vi "p2.vi"() -> ()   [LabVIEW 2023, in "d13.lvlib"]
uses:
  d13.lvlib
  AOC/AOC.lvlib
panel:
  out "XY Graph":cluster{i32, i32}[](graph)
  in  "Example":string="#.##..##.\n..#.##.#.\n##......#\n##......#\n..#.##.#.\n..##..##.\n#.#.##.#.\n\n#...##..#\n#....#..#\n..##..###\n#####.##.\n#####.##.\n..##..###\n#....#..#"
  in  "Example":bool=TRUE
  out "Answer":u64=5675
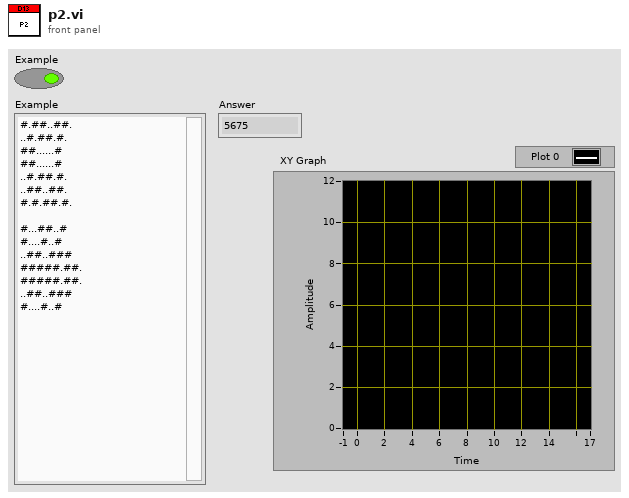
[diagram p1: front panel]
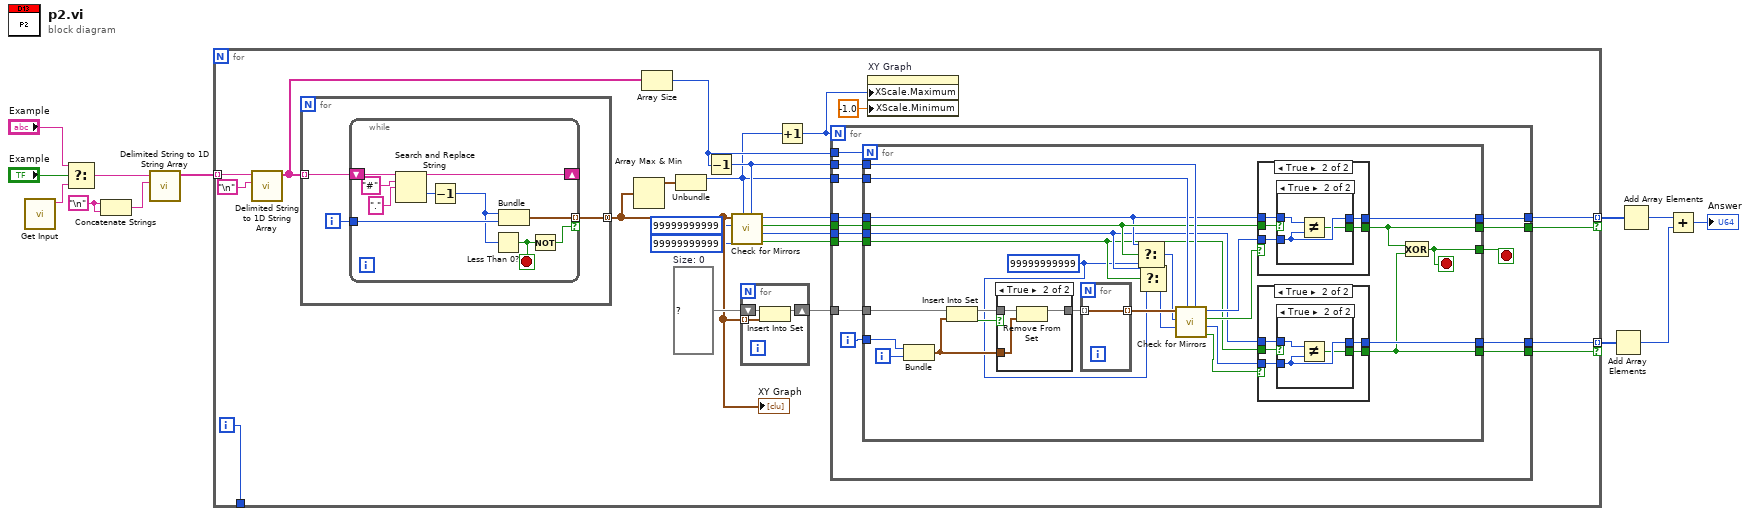
[diagram p0: block diagram]
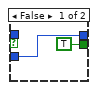
[diagram p3: hidden frame]
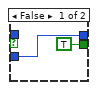
[diagram p5: hidden frame]
diagram:
  w5 = "\n"
  n1 = call "Get Input.vi"() -> ("Input"=w12:string)  [unwired: 11 in]
  n2 = Select(t="Example", s="Example", f=w12) -> (s? t:f=w8:string)
  n3 = Concatenate Strings(w5, w5) -> (w6:string)
  n4 = call <vilib>:"Delimited String to 1D String Array.vi"("delimiter"=w6, "delimited string"=w8) -> ("string array"=w7:string[])  [unwired: 9 in]
  n5 = for {
    tunnel: w7 -> [w35] mode=indexing
    tunnel: [w23] -> w9 mode=indexing if=w20
    tunnel: [w24] -> w4 mode=indexing if=w19
    tunnel: [w18] -> _
    i -> [w18]
    w31 = set{cluster{i32, i32}} {}  # Size: 0
    n6 = call <vilib>:"Delimited String to 1D String Array.vi"("delimiter"="\n", "delimited string"=w35) -> ("string array"=w32:string[])  [unwired: 9 in]
    n7 = for {
      tunnel: w32 -> [w110] mode=indexing
      tunnel: [w109] -> w17 mode=concatenating
      i -> [w108]
      n8 = while {
        tunnel: [w120] -> w109 mode=indexing if=w117
        tunnel: w108 -> [w119]
        shift-right: [w115] -> _
        shift-left: w110 -> [w116]
        stop <- w118 stop-if-true
        n9 = Search and Replace String(input string=w116, search string="#" ("search string/char (-)"), replace string="." ("replace string (\"\")")) -> (result string=w115:string, offset past replacement=w113:i32)  [unwired: 5 in, 2 out]
        n10 = Decrement(x=w113) -> (x-1=w112:i32)
        n11 = Less Than 0?(x=w112) -> (x < 0?=w118:bool)
        n12 = Bundle(w112, w119) -> (w120:cluster{i32, i32})  [unwired: 1 in]
        n13 = Not(x=w118) -> (.not. x?=w117:bool)
      }
    }
    "XY Graph" <- w17
    n14 = Array Max & Min(array=w17) -> (max value=w33:cluster{i32, i32})  [unwired: 3 out]
    n15 = Array Size(array=w32) -> (size(s)=w22:i32)
    n16 = Unbundle(w33) -> (w21:i32)  [unwired: 1 out]
    n17 = Decrement(x=w22) -> (x-1=w29:i32)
    n18 = call "Check for Mirrors.vi"("Ny"=w29, "Nx"=w21, "yPrev"=u64 99999999999, "xPrev"=u64 99999999999, "Rocks"=w17) -> ("Horizontal Mirror?"=w26:bool, "Mirrored Rows"=w27:u64, "Vertical Mirror?"=w25:bool, "Mirrored Columns"=w28:u64)  [unwired: 3 in]
    n19 = for {
      tunnel: w17 -> [w38] mode=indexing
      shift-right: [w36] -> w30
      shift-left: w31 -> [w37]
      n20 = Insert Into Set(10:w38, 11:w37) -> (3:w36:set{cluster{i32, i32}})  [unwired: 1 out]
    }
    n21 = Increment(x=w21) -> (x+1=w15:i32)
    n22 = for {
      N: w15 -> [_]
      tunnel: w28 -> [w50]
      tunnel: w25 -> [w48]
      tunnel: w27 -> [w49]
      tunnel: w26 -> [w47]
      tunnel: w29 -> [w42]
      tunnel: w30 -> [w52]
      tunnel: [w46] -> w23
      tunnel: [w45] -> w24
      tunnel: w21 -> [w43]
      tunnel: w22 -> [w41]
      tunnel: [w40] -> w20
      tunnel: [w39] -> w19
      i -> [w51]
      stop <- w44 stop-if-true
      n23 = for {
        N: w41 -> [_]
        tunnel: w52 -> [w78]
        tunnel: w51 -> [w76]
        tunnel: w50 -> [w58]
        tunnel: w49 -> [w55]
        tunnel: w48 -> [w59]
        tunnel: w47 -> [w54]
        tunnel: [w68] -> w46
        tunnel: [w67] -> w45
        tunnel: [w66] -> w44
        tunnel: w43 -> [w65]
        tunnel: w42 -> [w62]
        tunnel: [w61] -> w40
        tunnel: [w60] -> w39
        i -> [w77]
        stop <- w66 stop-if-true
        w53 = u64 99999999999 ("yPrev")
        n24 = Bundle(w76, w77) -> (w74:cluster{i32, i32})  [unwired: 1 in]
        n25 = Insert Into Set(10:w74, 11:w78) -> (2:w73:bool, 3:w75:set{cluster{i32, i32}})
        n26 = case shown="True" w73 {
          tunnel: w75 -> [w104 w107]
          tunnel: w74 -> [_ w106]
          tunnel: [w104 w105] -> w72
          frame False {
          }
          frame True {
            n27 = Remove From Set(10:w106, 11:w107) -> (3:w105:set{cluster{i32, i32}})  [unwired: 1 out]
          }
        }
        n28 = for {
          tunnel: w72 -> [w103] mode=indexing
          tunnel: [w103] -> w71 mode=indexing
        }
        n29 = Select(t=w58, s=w59, f=w53) -> (s? t:f=w57:u64)
        n30 = Select(t=w55, s=w54, f=w53) -> (s? t:f=w56:u64)
        n31 = call "Check for Mirrors.vi"("Ny"=w62, "Nx"=w65, "yPrev"=w56, "xPrev"=w57, "Rocks"=w71) -> ("Horizontal Mirror?"=w63:bool, "Mirrored Rows"=w69:u64, "Vertical Mirror?"=w64:bool, "Mirrored Columns"=w70:u64)  [unwired: 3 in]
        n32 = case shown="True" w64 {
          selector: w64 -> [w92 _]
          tunnel: w58 -> [_ w95]
          tunnel: w59 -> [_ w97]
          tunnel: w70 -> [w91 w96]
          tunnel: [w91 w94] -> w68
          tunnel: [w92 w93] -> w61
          frame False {
          }
          frame True {
            n33 = case shown="True" w97 {
              tunnel: w96 -> [w99 w101]
              tunnel: w95 -> [_ w102]
              tunnel: [w99 w101] -> w94
              tunnel: [TRUE w100] -> w93
              frame False {
              }
              frame True {
                n34 = Not Equal?(x=w102, y=w101) -> (x != y?=w100:bool)
              }
            }
          }
        }
        n35 = case shown="True" w63 {
          selector: w63 -> [w80 _]
          tunnel: w55 -> [_ w83]
          tunnel: w54 -> [_ w85]
          tunnel: w69 -> [w79 w84]
          tunnel: [w79 w82] -> w67
          tunnel: [w80 w81] -> w60
          frame False {
          }
          frame True {
            n36 = case shown="True" w85 {
              tunnel: w84 -> [w87 w89]
              tunnel: w83 -> [_ w90]
              tunnel: [w87 w89] -> w82
              tunnel: [TRUE w88] -> w81
              frame False {
              }
              frame True {
                n37 = Not Equal?(x=w90, y=w89) -> (x != y?=w88:bool)
              }
            }
          }
        }
        n38 = Exclusive Or(1:w60, 2:w61) -> (0:w66:bool)
      }
    }
    n39 = property on="XY Graph" class="XYGraph (strict)"("XScale.Maximum"=w15, "XScale.Minimum"=-1.0 ("X Scale.Range:Minimum")) -> ()  [unwired: 2 in, 2 out]
  }
  n40 = Add Array Elements(numeric array=w4) -> (sum=w3:u64)
  n41 = Add Array Elements(numeric array=w9) -> (sum=w2:u64)
  n42 = Add(x=w2, y=w3) -> (x+y=→"Answer":u64)
